vi "ServiceProviderExample.vi"() -> ()   [LabVIEW 2012]
uses:
  <userlib>/ROS for LabVIEW Software/ROS/MessageParsing/std_msgs/subs/parse_i64_scalar.vi
  <userlib>/ROS for LabVIEW Software/ROS/MessageBuilding/std_msgs/subs/i64Scalar.vi
panel:
  out "y":i64
  out "x":i64
  in  "stop":bool
  out "x+y":i64
  out "Request":string
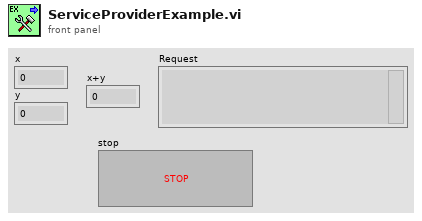
[diagram p1: front panel]
types:
  T1 = typedef "_ROSControl.ctl" = cluster{"topic port":u16, "Node":string, "topic":string, "type":string, "node port":u16, "error ":errorcluster, "Direction":T2, "Update (ms)":u16, "FIFO size":u16}
  T2 = typedef "_ROSDirection.ctl" = enum16{"Node", "Publisher", "Subscriber", "ServiceClient", "ServiceProvider"}
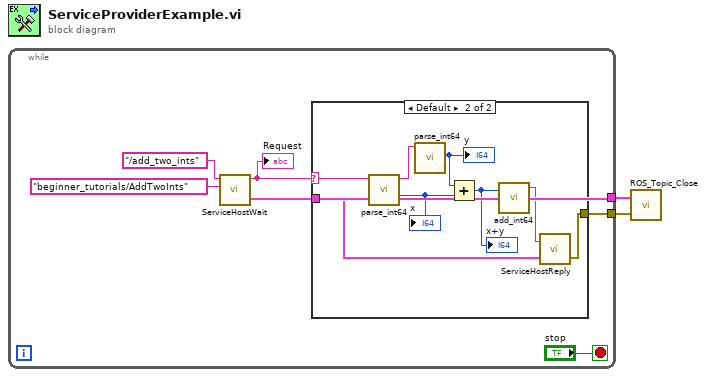
[diagram p0: block diagram]
diagram:
  n1 = while {
    tunnel: [w4] -> w2
    tunnel: [w3] -> w1
    stop <- "stop" stop-if-true
    n2 = call <userlib>:"ServiceHostWait.vi"("Topic"="/add_two_ints", "Type"="beginner_tutorials/AddTwoInts") -> ("Request"=w7:string, "Service ROS info out"=w4:T1)  [unwired: 3 in]
    "Request" <- w7
    n3 = case shown="Default" w7 {
      selector: w7 -> [_ w15]
      tunnel: w4 -> [_ w16]
      tunnel: [_ w9] -> w3
      frame "" {
      }
      frame Default {
        n4 = call-poly <userlib>:"parse_int64.vi"("msg in"=w15) -> ("number"=w12:i64, "msg out"=w14:string)  [unwired: 4 in, 1 out]
        "x" <- w12
        n5 = call-poly <userlib>:"parse_int64.vi"("msg in"=w14) -> ("number"=w13:i64)  [unwired: 4 in, 2 out]
        "y" <- w13
        n6 = Add(x=w13, y=w12) -> (x+y=w11:i64)
        "x+y" <- w11
        n7 = call-poly <userlib>:"add_int64.vi"("Numeric"=w11) -> ("msg out"=w10:string)  [unwired: 4 in]
        n8 = call <userlib>:"ServiceHostReply.vi"("Service ROS info in"=w16, "Reply"=w10) -> ("error out"=w9:errorcluster)  [unwired: 2 in]
      }
    }
  }
  n9 = call <userlib>:"ROS_Topic_Close.vi"("error in"=w1, "ROS in"=w2) -> ()  [unwired: 2 in, 1 out]
